vi "Divide Rational Polynomials (DBL).vi"(4 "threshold type":T1 items=["Absolute Value", "Relative Value"], 6 "threshold":dbl, 8 "Denominator 2":dbl[](array[numeric]) min=0.0 max=127.0 format="%#.2g", 9 "Numerator 2":dbl[](array[numeric]) min=0.0 max=127.0 format="%#.2g", 10 "Denominator 1":dbl[](array[numeric]) min=0.0 max=127.0 format="%#.2g", 11 "Numerator 1":dbl[](array[numeric]) min=0.0 max=127.0 format="%#.2g") -> (0 "error":i32, 2 "Denominator Out":dbl[](array[numeric]) min=0.0 max=127.0 format="%#.2g", 3 "Numerator Out":dbl[](array[numeric]) min=0.0 max=127.0 format="%#.2g")   [LabVIEW 2010, in "NI_AALPro.lvlib"]
doc: "Divides rational polynomial G1 by rational polynomial G2. The data types you wire to the <B>Numerator 1</B>, <B>Denominator 1</B>, <B>Numerator 2</B>, and <B>Denominator 2</B> inputs determine the polymorphic instance to use."
uses:
  NI_AALPro.lvlib
  Remove Zero Threshold Type.ctl
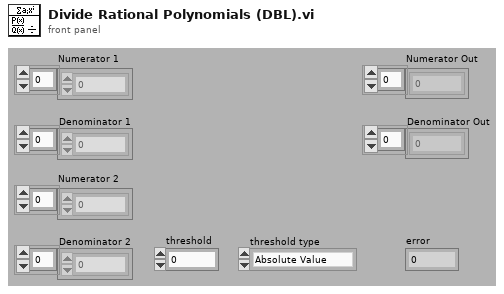
[diagram p1: front panel]
types:
  T1 = typedef "NI_AALPro.lvlib/Remove Zero Threshold Type.ctl" = u16
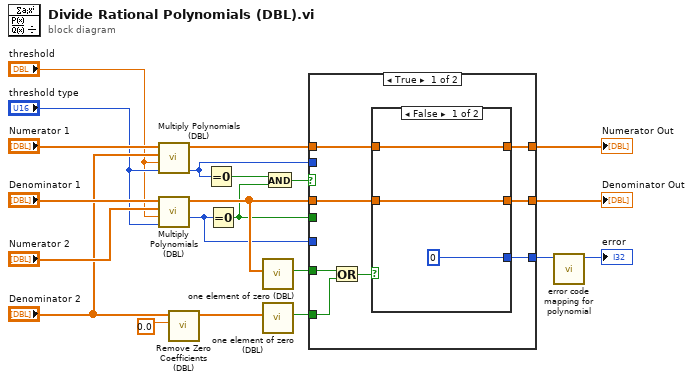
[diagram p0: block diagram]
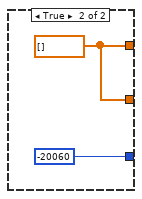
[diagram p2: hidden frame]
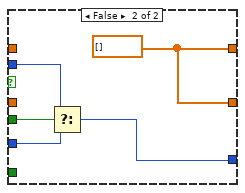
[diagram p3: hidden frame]
diagram:
  n1 = call "Multiply Polynomials (DBL).vi"("threshold type"="threshold type", "threshold"="threshold", "Q(x)"="Denominator 2", "P(x)"="Numerator 1") -> ("error"=w7:i32, "P(x)*Q(x)"=w18:dbl[])  [unwired: 6 in]
  n2 = call "Multiply Polynomials (DBL).vi"("threshold type"="threshold type", "threshold"="threshold", "Q(x)"="Numerator 2", "P(x)"="Denominator 1") -> ("error"=w4:i32, "P(x)*Q(x)"=w12:dbl[])  [unwired: 6 in]
  n3 = call "Remove Zero Coefficients (DBL).vi"("threshold"=0.0, "P(x) In"="Denominator 2") -> ("P(x) Out"=w13:dbl[])  [unwired: 7 in, 2 out]
  n4 = Equal To 0?(x=w7) -> (x = 0?=w6:bool)
  n5 = Equal To 0?(x=w4) -> (x = 0?=w3:bool)
  n6 = call "one element of zero (DBL).vi"("Array in"=w12) -> ("equal [0]?"=w11:bool)  [unwired: 10 in]
  n7 = call "one element of zero (DBL).vi"("Array in"=w13) -> ("equal [0]?"=w10:bool)  [unwired: 10 in]
  n8 = And(x=w6, y=w3) -> (x .and. y?=w5:bool)
  n9 = case shown="True" w5 {
    tunnel: w18 -> [w28 _]
    tunnel: w12 -> [w29 _]
    tunnel: [w27 w39] -> w17
    tunnel: [w26 w39] -> w16
    tunnel: [w25 w36] -> w9
    tunnel: w11 -> [w23 _]
    tunnel: w10 -> [w22 _]
    tunnel: w7 -> [_ w38]
    tunnel: w4 -> [_ w37]
    tunnel: w3 -> [_ w35]
    frame True {
      n10 = Or(x=w23, y=w22) -> (x .or. y?=w24:bool)
      n11 = case shown="False" w24 {
        tunnel: w29 -> [w30 _]
        tunnel: w28 -> [w31 _]
        tunnel: [0 -20060 ("divide by zero")] -> w25
        tunnel: [w31 w33] -> w27
        tunnel: [w30 w33] -> w26
        frame False {
        }
        frame True {
          w33 = dbl[] [] ("BDL")
        }
      }
    }
    frame False {
      w39 = dbl[] [] ("BDL")
      n12 = Select(t=w38, s=w35, f=w37) -> (s? t:f=w36:i32)
    }
  }
  "Numerator Out" <- w17
  "Denominator Out" <- w16
  n13 = call "error code mapping for polynomial.vi"("error in"=w9) -> ("error out"=→"error":i32)  [unwired: 10 in]
